vi "Factor de escala.vi"(11 "Knob":dbl) -> (3 "Numeric":dbl)   [LabVIEW 2020]
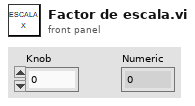
[diagram p1: front panel]
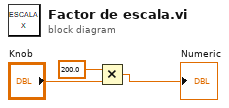
[diagram p0: block diagram]
diagram:
  n1 = Multiply(x=200.0, y="Knob") -> (x*y=→"Numeric":dbl)
